vi "Start connection wrapper test.vi"() -> ()   [LabVIEW 2022 SP3]
uses:
  <vilib>/addons/zeromq/socket_type.ctl
  <vilib>/addons/zeromq/zmq_context.lvclass
  <vilib>/addons/zeromq/zmq_socket.lvclass
  <vilib>/addons/zeromq/zeromq.lvlib
panel:
  out "Standalone":bool
  in  "error in":errorcluster
  out "resulting string":string
  out "error out":errorcluster
  in  "Instrument":string
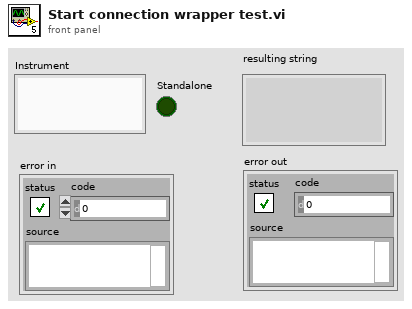
[diagram p1: front panel]
types:
  T1 = typedef "zeromq.lvlib/socket_type.ctl" = enum8{"ZMQ_PAIR", "ZMQ_PUB", "ZMQ_SUB", "ZMQ_REQ", "ZMQ_REP", "ZMQ_DEALER", "ZMQ_ROUTER", "ZMQ_PULL", "ZMQ_PUSH", "ZMQ_XPUB", "ZMQ_XSUB", "ZMQ_STREAM", "ZMQ_SERVER", "ZMQ_CLIENT", "ZMQ_RADIO", "ZMQ_DISH", "ZMQ_GATHER", "ZMQ_SCATTER", "ZMQ_DGRAM"}
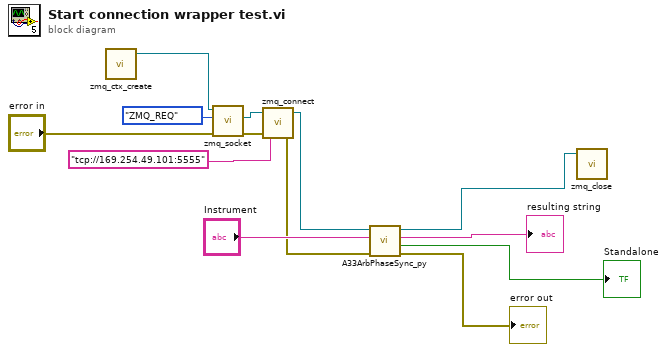
[diagram p0: block diagram]
diagram:
  n1 = call <vilib>:"zmq_ctx_create.vi"() -> ("context out"=w10:refnum<class "zmq_context.lvclass">)  [unwired: 4 in, 1 out]
  n2 = call <vilib>:"zmq_socket.vi"("error in"="error in", "socket type"=socket_type."ZMQ_REQ", "context in"=w10) -> ("error out"=w6:errorcluster, "socket out"=w7:refnum<class "zmq_socket.lvclass">)  [unwired: 2 in, 1 out]
  n3 = call <vilib>:"zmq_connect.vi"("error in"=w6, "endpoint"="tcp://169.254.49.101:5555", "socket in"=w7) -> ("error out"=w3:errorcluster, "socket out"=w5:refnum<class "zmq_socket.lvclass">)  [unwired: 1 in]
  n4 = call "A33ArbPhaseSync_py.vi"("error in (no error)"=w3, "Instrument"="Instrument", "socket in"=w5) -> ("error out"=→"error out":errorcluster, "Standalone"=→"Standalone":bool, "resulting string"=→"resulting string":string, "socket out"=w2:refnum<class "zmq_socket.lvclass">)  [unwired: 5 in]
  n5 = call <vilib>:"zmq_close.vi"("socket"=w2) -> ()  [unwired: 4 in, 1 out]
